vi "Test Find Class from Path Prod Namespace.vi"(8 "error in (no error)":errorcluster, 11 "Test Finder Test in":refnum<class "Test Finder Test.lvclass">) -> (0 "error out":errorcluster, 3 "Test Finder Test out":refnum<class "Test Finder Test.lvclass">)   [LabVIEW 2020, in "LUnit Tests.lvlib" / "Test Finder Test.lvclass"]
uses:
  Test Finder Test.lvclass
  C:/Program Files (x86)/National Instruments/LabVIEW 2020/vi.lib/Astemes/LUnit/Test Case.lvclass
  source/Framework/Helper Classes/Test Finder/Test Finder.lvclass
  <vilib>/Astemes/LUnit/Test Case.lvclass/Test Case.ctl
  <vilib>/Astemes/LUnit/LUnit Assertion Result.lvclass/LUnit Assertion Result.ctl
  <vilib>/Astemes/LUnit/LUnit Test Case Result.lvclass/LUnit Test Case Result.ctl
  <vilib>/Astemes/LUnit/LUnit Method Result.lvclass/LUnit Method Result.ctl
  <vilib>/Astemes/LUnit/Palette/Fail.vi
  <vilib>/Astemes/LUnit/Palette/Pass.vi
  <vilib>/Astemes/LUnit/Set Assertion Type.vi
  <vilib>/Astemes/LUnit/Add test result.vi
  <vilib>/Astemes/LUnit/LUnit Write Passed.vi
  <vilib>/Astemes/LUnit/LUnit Write Message.vi
  <vilib>/Astemes/LUnit/LUnit Write Description.vi
  <vilib>/Astemes/LUnit/LUnit Write Assertion Type.vi
  <vilib>/Astemes/LUnit/LUnit Record Assertion Result.vi
  <vilib>/Astemes/LUnit/LUnit Aggregate Assertion Results.vi
  <vilib>/Astemes/LUnit/Assertion Result/LUnit Read Status.vi
  <vilib>/Astemes/LUnit/LUnit Read Message.vi
  <vilib>/Astemes/LUnit/LUnit Read Description.vi
  <vilib>/Astemes/LUnit/Method Result/LUnit Merge Status.vi
  <vilib>/Astemes/LUnit/LUnit Concatenate result strings.vi
  <vilib>/Astemes/LUnit/LUnit Assertion Result.lvclass
  <vilib>/Astemes/LUnit/Test Case.lvclass
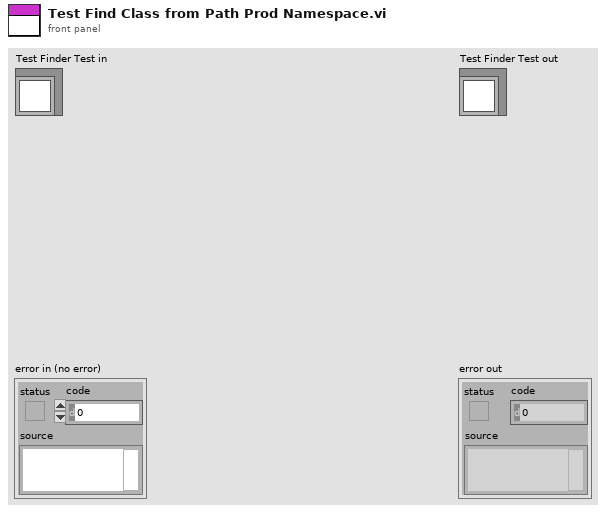
[diagram p1: front panel]
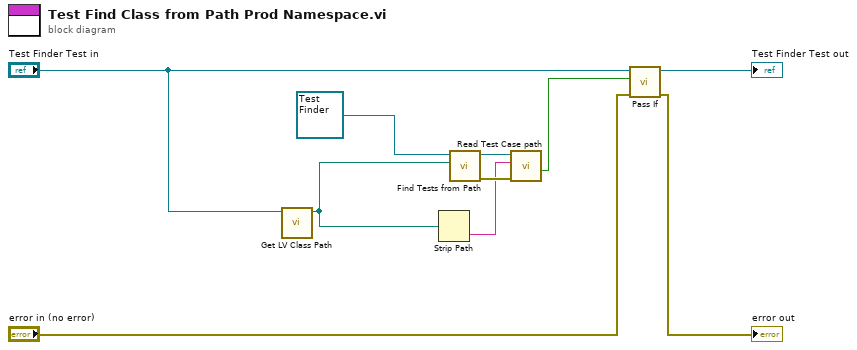
[diagram p0: block diagram]
diagram:
  n1 = call <vilib>:"Get LV Class Path.vi"("object"="Test Finder Test in") -> ("class path"=w4:path)  [unwired: 9 in, 1 out]
  n2 = Strip Path(path=w4) -> (name=w3:string)  [unwired: 1 out]
  n3 = call-dynamic "Find Tests from Path.vi"("Project or Class Path"=w4, "Test Case Finder In"=refnum<class "Test Finder.lvclass"> refnum) -> ("error out"=w6:errorcluster, "Test Case Finder Out"=w7:refnum<class "Test Finder.lvclass">)  [unwired: 8 in]
  n4 = call "Read Test Case path.vi"("error in (no error)"=w6, "Test Case Name"=w3, "Test Case Finder In"=w7) -> ("found?"=w2:bool)  [unwired: 5 in, 3 out]
  n5 = call <vilib>:"Pass If.vi"("error in (no error)"="error in (no error)", "Pass?"=w2, "LUnit Test Case In"="Test Finder Test in") -> ("error out"=→"error out":errorcluster, "LUnit Test Case Out"=→"Test Finder Test out":refnum<class "Test Finder Test.lvclass">)  [unwired: 7 in]
